vi "Config Write Auton Globals.vi"(11 "refnum":T1) -> (3 "refnum 2":T1)   [LabVIEW 2012]
uses:
  <vilib>/Utility/config.llb/Config Data RefNum.ctl
  Auton Globals.vi
  <vilib>/Utility/config.llb/Write Key (Double).vi
  <vilib>/Utility/config.llb/NI_LVConfig.lvlib
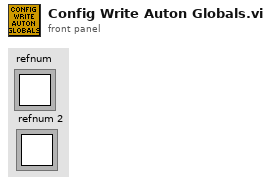
[diagram p1: front panel]
types:
  T1 = typedef "NI_LVConfig.lvlib/Config Data RefNum.ctl" = refnum<k1>
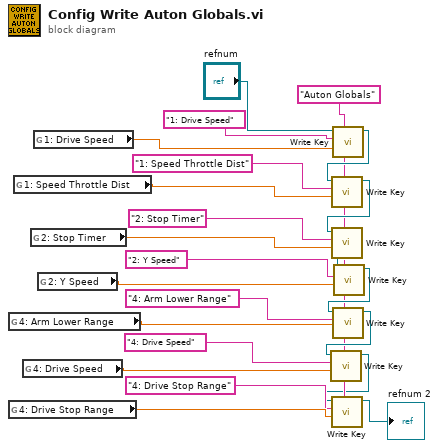
[diagram p0: block diagram]
diagram:
  w10 = "Auton Globals"
  n1 = global read "Auton Globals.vi" "4: Arm Lower Range"() -> (w7:dbl)
  n2 = global read "Auton Globals.vi" "4: Drive Stop Range"() -> (w9:dbl)
  n3 = global read "Auton Globals.vi" "1: Speed Throttle Dist"() -> (w4:dbl)
  n4 = global read "Auton Globals.vi" "4: Drive Speed"() -> (w8:dbl)
  n5 = global read "Auton Globals.vi" "2: Stop Timer"() -> (w5:dbl)
  n6 = global read "Auton Globals.vi" "1: Drive Speed"() -> (w11:dbl)
  n7 = global read "Auton Globals.vi" "2: Y Speed"() -> (w6:dbl)
  n8 = call-poly <vilib>:"Write Key.vi"("section"=w10, "value"=w11, "key"="1: Drive Speed", "refnum"="refnum") -> ("refnum out"=w22:T1)  [unwired: 5 in, 2 out]
  n9 = call-poly <vilib>:"Write Key.vi"("section"=w10, "value"=w4, "key"="1: Speed Throttle Dist", "refnum"=w22) -> ("refnum out"=w21:T1)  [unwired: 5 in, 2 out]
  n10 = call-poly <vilib>:"Write Key.vi"("section"=w10, "value"=w5, "key"="2: Stop Timer", "refnum"=w21) -> ("refnum out"=w20:T1)  [unwired: 5 in, 2 out]
  n11 = call-poly <vilib>:"Write Key.vi"("section"=w10, "value"=w6, "key"="2: Y Speed", "refnum"=w20) -> ("refnum out"=w19:T1)  [unwired: 5 in, 2 out]
  n12 = call-poly <vilib>:"Write Key.vi"("section"=w10, "value"=w7, "key"="4: Arm Lower Range", "refnum"=w19) -> ("refnum out"=w18:T1)  [unwired: 5 in, 2 out]
  n13 = call-poly <vilib>:"Write Key.vi"("section"=w10, "value"=w8, "key"="4: Drive Speed", "refnum"=w18) -> ("refnum out"=w2:T1)  [unwired: 5 in, 2 out]
  n14 = call-poly <vilib>:"Write Key.vi"("section"=w10, "value"=w9, "key"="4: Drive Stop Range", "refnum"=w2) -> ("refnum out"=→"refnum 2":T1)  [unwired: 5 in, 2 out]
